vi "1欢迎界面1.vi"() -> ()   [LabVIEW 2016]
panel:
  out "error constant 2":errorcluster caption="error constant"
  in  "error constant":errorcluster
  # "欢迎关注：\n                             \n\n  Labview学习日记"
  # "版本：1.0\nCopyright@2019lover"
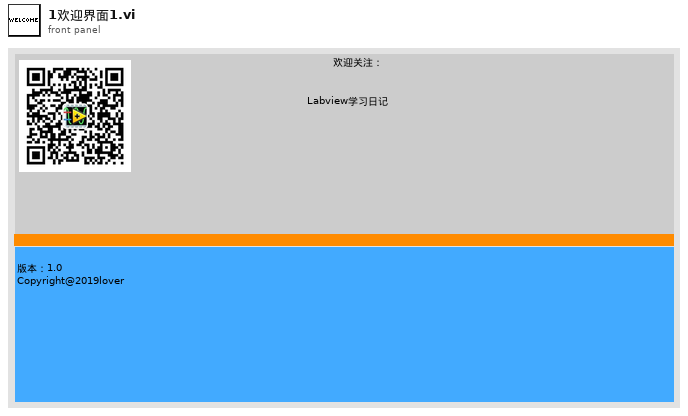
[diagram p1: front panel]
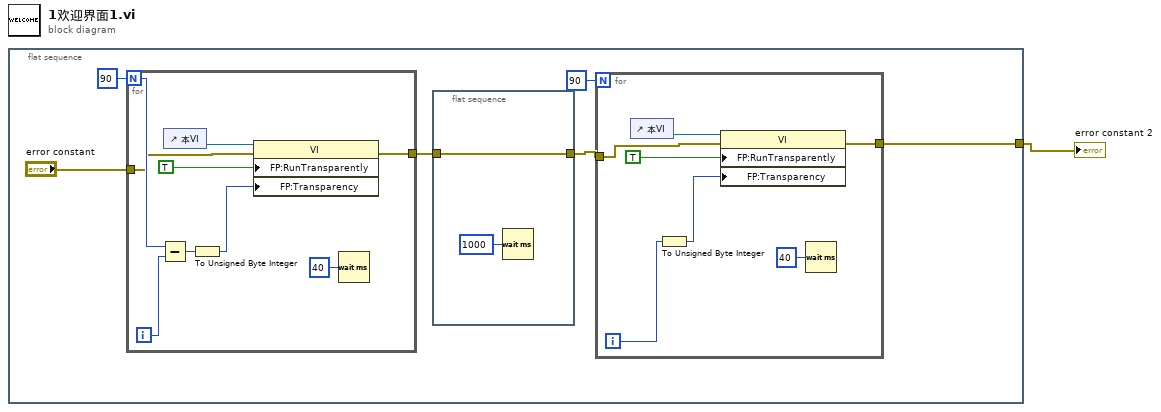
[diagram p0: block diagram]
diagram:
  n1 = flat-sequence {
    tunnel: [w2] -> w1
    frame #0 {
      n2 = for {
        N: 90 -> [w19]
        tunnel: "error constant" -> [w18]
        tunnel: [w17] -> w6
        i -> [w20]
        n3 = Subtract(x=w19, y=w20) -> (x-y=w25:i32)
        n4 = control-ref of="本VI"() -> (w23:refnum<vi>)
        n5 = To Unsigned Byte Integer(number=w25) -> (unsigned 8bit integer=w21:u8)
        n6 = property class="VI"(reference=w23, error in=w18, "FP:RunTransparently"=TRUE, "FP:Transparency"=w21) -> (error out=w17:errorcluster)  [unwired: 1 out]
        n7 = Wait (ms)(milliseconds to wait=u32 40 ("等待时间（毫秒）")) -> ()  [unwired: 1 out]
      }
      n8 = flat-sequence {
        tunnel: w6 -> [w16]
        tunnel: [w16] -> w7
        frame #0 {
          n9 = Wait (ms)(milliseconds to wait=u32 1000 ("等待时间（毫秒）")) -> ()  [unwired: 1 out]
        }
      }
      n10 = for {
        N: 90 -> [_]
        tunnel: w7 -> [w9]
        tunnel: [w8] -> w2
        i -> [w10]
        n11 = control-ref of="本VI"() -> (w13:refnum<vi>)
        n12 = To Unsigned Byte Integer(number=w10) -> (unsigned 8bit integer=w11:u8)
        n13 = property class="VI"(reference=w13, error in=w9, "FP:RunTransparently"=TRUE, "FP:Transparency"=w11) -> (error out=w8:errorcluster)  [unwired: 1 out]
        n14 = Wait (ms)(milliseconds to wait=u32 40 ("等待时间（毫秒）")) -> ()  [unwired: 1 out]
      }
    }
  }
  "error constant 2" <- w1
